vi "mxwScript_API_Option_UniquificationObjects.vi"(8 "error in (no error)":errorcluster, 10 "uniquificationObjects":string[](array[string])=["FlatSequence", "Structure", "Constant", "ControlTerminal"], 11 "options in":T1[](array[typedef])) -> (0 "error out":errorcluster, 3 "options out":T1[](array[typedef]))   [LabVIEW 2020]
doc: "Sets the object types uniquified during code generation."
uses:
  codeGenAPISupport.llb/cgAPI_mxwScript_OptionData.ctl
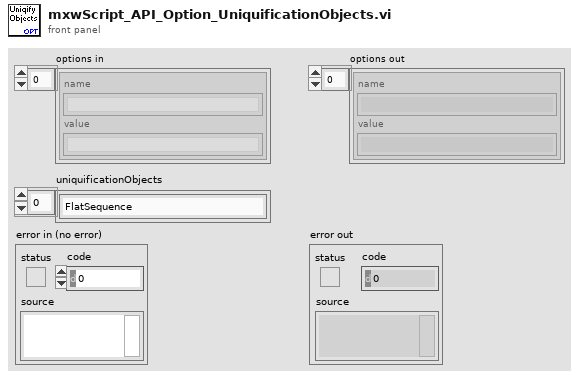
[diagram p1: front panel]
types:
  T1 = typedef "cgAPI_mxwScript_OptionData.ctl" = cluster{"name":string, "value":string}
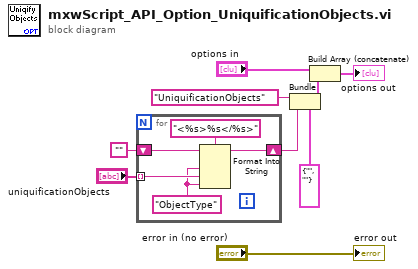
[diagram p0: block diagram]
diagram:
  n1 = for {
    tunnel: "uniquificationObjects" -> [w12] mode=indexing
    shift-right: [w11] -> w1
    shift-left: "" -> [w14]
    w10 = "ObjectType" ("format string")
    n2 = Format Into String(format string="<%s>%s</%s>", initial string=w14, w10, w12, w10) -> (resulting string=w11:string)  [unwired: 1 in, 1 out]
  }
  n3 = Bundle(cluster=T1 {"name"="", "value"=""} ("optionData"), "name"="UniquificationObjects", "value"=w1) -> (w7:T1)
  n4 = Build Array (concatenate)("options in", w7) -> (→"options out":T1[])
  "error out" <- "error in (no error)"
